vi "Initialize Attributes.vi"(8 "error in (no error)":errorcluster, 10 "Attribute Data":variant, 11 "CS++BaseActor in":refnum<class "CS++BaseActor.lvclass">) -> (0 "error out":errorcluster, 2 "Found?":bool, 3 "CS++BaseActor out":refnum<class "CS++BaseActor.lvclass">)   [LabVIEW 2014, in "CS++BaseActor.lvlib" / "CS++BaseActor.lvclass"]
doc: "Initialize object attribute.\n\nUnique resources should be allocated elsewhere!"
uses:
  CS++BaseActor.lvclass
  CS++BaseActor.lvclass/CS++BaseActor.ctl
  Libraries/Utilities/CS++Utilities.lvlib
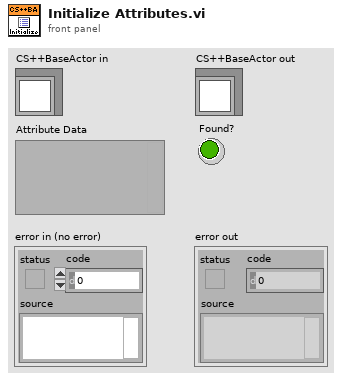
[diagram p1: front panel]
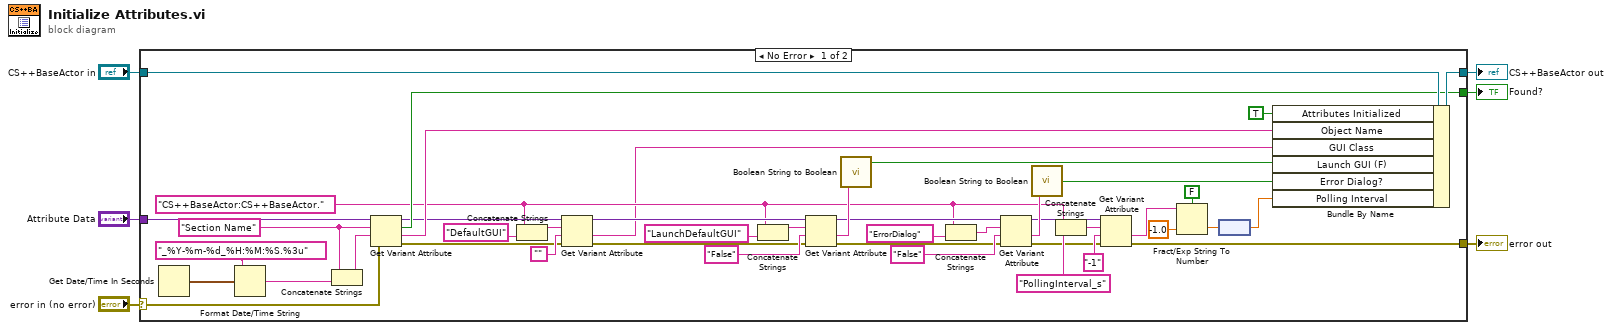
[diagram p0: block diagram]
diagram:
  n1 = case shown="No Error" "error in (no error)" {
    selector: "error in (no error)" -> [w44 w52]
    tunnel: [w11 w52] -> w1
    tunnel: [w49 w51] -> w5
    tunnel: "CS++BaseActor in" -> [w50 w51]
    tunnel: "Attribute Data" -> [w48 _]
    tunnel: [w33 _] -> w3
    frame No Error {
      w13 = "CS++BaseActor:CS++BaseActor."
      w42 = "Section Name" ("name")
      n2 = Get Date/Time In Seconds() -> (seconds since 1Jan1904=w47:timestamp)
      n3 = Format Date/Time String(time format string (%c)="_%Y-%m-%d_%H:%M:%S.%3u", seconds (now)=w47) -> (date/time string=w45:string)  [unwired: 1 in]
      n4 = Concatenate Strings(w42, w45) -> (w43:string)
      n5 = Get Variant Attribute(Variant=w48, name=w42, default value (empty Variant)=w43, error in=w44) -> (duplicate Variant=w31:variant, found=w33:bool, value=w32:string, error out=w28:errorcluster)
      n6 = Concatenate Strings(w13, "DefaultGUI") -> (w41:string)
      n7 = Get Variant Attribute(Variant=w31, name=w41, default value (empty Variant)="", error in=w28) -> (duplicate Variant=w34:variant, value=w7:string, error out=w36:errorcluster)  [unwired: 1 out]
      n8 = Concatenate Strings(w13, "LaunchDefaultGUI") -> (w37:string)
      n9 = Get Variant Attribute(Variant=w34, name=w37, default value (empty Variant)="False", error in=w36) -> (duplicate Variant=w21:variant, value=w35:string, error out=w10:errorcluster)  [unwired: 1 out]
      n10 = call "Boolean String to Boolean.vi"("T/F String"=w35) -> ("Value"=w29:bool)
      n11 = Concatenate Strings(w13, "ErrorDialog") -> (w25:string)
      n12 = Get Variant Attribute(Variant=w21, name=w25, default value (empty Variant)="False", error in=w10) -> (duplicate Variant=w9:variant, value=w26:string, error out=w14:errorcluster)  [unwired: 1 out]
      n13 = call "Boolean String to Boolean.vi"("T/F String"=w26) -> ("Value"=w22:bool)
      n14 = Concatenate Strings(w13, "PollingInterval_s" ("string")) -> (w17:string)
      n15 = Get Variant Attribute(Variant=w9, name=w17, default value (empty Variant)="-1" ("string"), error in=w14) -> (value=w18:string, error out=w11:errorcluster)  [unwired: 2 out]
      n16 = Fract/Exp String To Number(use system decimal point (T)=FALSE, string=w18, default (0 dbl)=-1.0 ("default (0 DBL)")) -> (number=w20:dbl)  [unwired: 1 in, 1 out]
      n17 = node(w20) -> (w12:dbl[unit])
      n18 = Bundle By Name(cluster=w50, "Attributes Initialized"=TRUE, "Object Name"=w32, "GUI Class"=w7, "Launch GUI (F)"=w29, "Error Dialog?"=w22, "Polling Interval"=w12) -> (w49:refnum<class "CS++BaseActor.lvclass">)
    }
    frame Error {
    }
  }
  "error out" <- w1
  "CS++BaseActor out" <- w5
  "Found?" <- w3
